vi "addres.vi"() -> ()   [LabVIEW 2017]
panel:
  out "number":string
  out "color":string
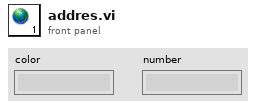
[diagram p1: front panel]
diagram:
